vi "TimeShiftData.vi"(3 "output cluster":T1, 4 "Array In":i16[][](array[numeric])) -> (0 "Array Out":i16[][](array[numeric]))   [LabVIEW 2022 SP3]
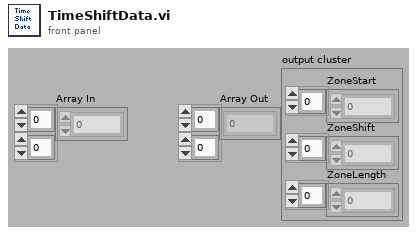
[diagram p1: front panel]
types:
  T1 = cluster{"ZoneStart":sgl[], "ZoneShift":sgl[], "ZoneLength":sgl[]}
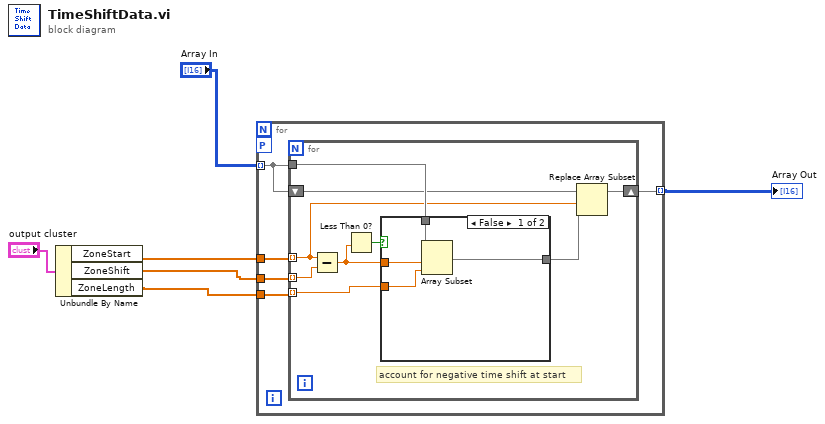
[diagram p0: block diagram]
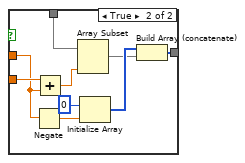
[diagram p2: hidden frame]
diagram:
  n1 = Unbundle By Name("output cluster") -> ("ZoneStart"=w3:sgl[], "ZoneShift"=w2:sgl[], "ZoneLength"=w1:sgl[])
  n2 = for {
    tunnel: "Array In" -> [w7] mode=indexing
    tunnel: w3 -> [w11]
    tunnel: w2 -> [w10]
    tunnel: w1 -> [w9]
    workers-P: _ -> [_]
    tunnel: [w8] -> w5 mode=indexing
    n3 = for {
      tunnel: w11 -> [w13] mode=indexing
      tunnel: w9 -> [w20] mode=indexing
      tunnel: w10 -> [w19] mode=indexing
      tunnel: w7 -> [w16]
      shift-right: [w15] -> w8
      shift-left: w7 -> [w14]
      # "account for negative time shift at start"
      n4 = Subtract(x=w13, y=w19) -> (x-y=w17:sgl)
      n5 = Less Than 0?(x=w17) -> (x < 0?=w18:bool)
      n6 = case shown="False" w18 {
        tunnel: w16 -> [w24 w32]
        tunnel: w20 -> [w22 w33]
        tunnel: [w23 w27] -> w12
        tunnel: w17 -> [w21 w30]
        frame False {
          n7 = Array Subset(array=w24, index=w21, length=w22) -> (w23:i16[])
        }
        frame True {
          n8 = Negate(x=w30) -> (-x=w25:sgl)
          n9 = Add(x=w33, y=w30) -> (x+y=w26:sgl)
          n10 = Array Subset(array=w32, length=w26) -> (w28:i16[])  [unwired: 1 in]
          n11 = Initialize Array(i16 0, w25) -> (w29:i16[])
          n12 = Build Array (concatenate)(w29, w28) -> (w27:i16[])
        }
      }
      n13 = Replace Array Subset(array=w14, new element=w12, index=w13) -> (w15:i16[])
    }
  }
  "Array Out" <- w5
